vi "integrate_resonance_multifunctional.vi"(0 "integration cluster in":T1, 2 "integration iterations per pixel":u32, 3 "number of pixels":u32, 5 "sampling values in":T2, 7 "choose TAG slice?":bool, 9 "iteration counter in":u32, 11 "pixel counter in":u32, 12 "pick first TAG slice":u32, 13 "pick lastTAG slice":u32, 14 "xy view?":bool) -> (4 "integration cluster out":T1, 6 "iteration counter out":u32, 10 "finished?":bool, 15 "pixel counter out":u32)   [LabVIEW 2010]
uses:
  common_typedefs/channels_cluster.ctl
  integration_cluster.ctl
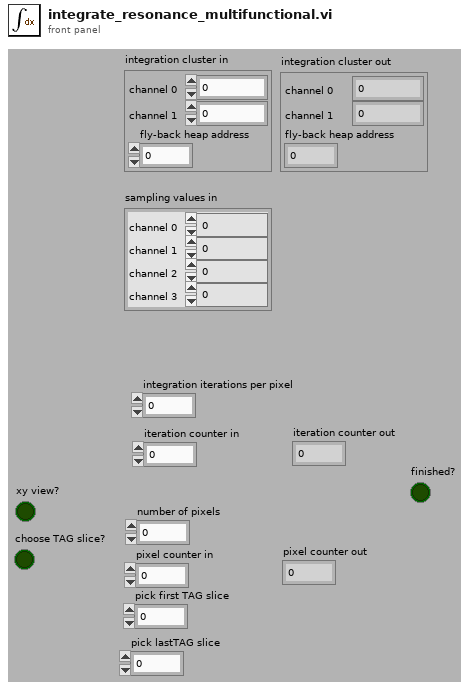
[diagram p1: front panel]
types:
  T1 = typedef "integration_cluster.ctl" = cluster{"channel 0":u32, "channel 1":u32, "fly-back heap address":u32}
  T2 = typedef "channels_cluster.ctl" = cluster{"channel 0":u32, "channel 1":u32, "channel 2":u32, "channel 3":u32}
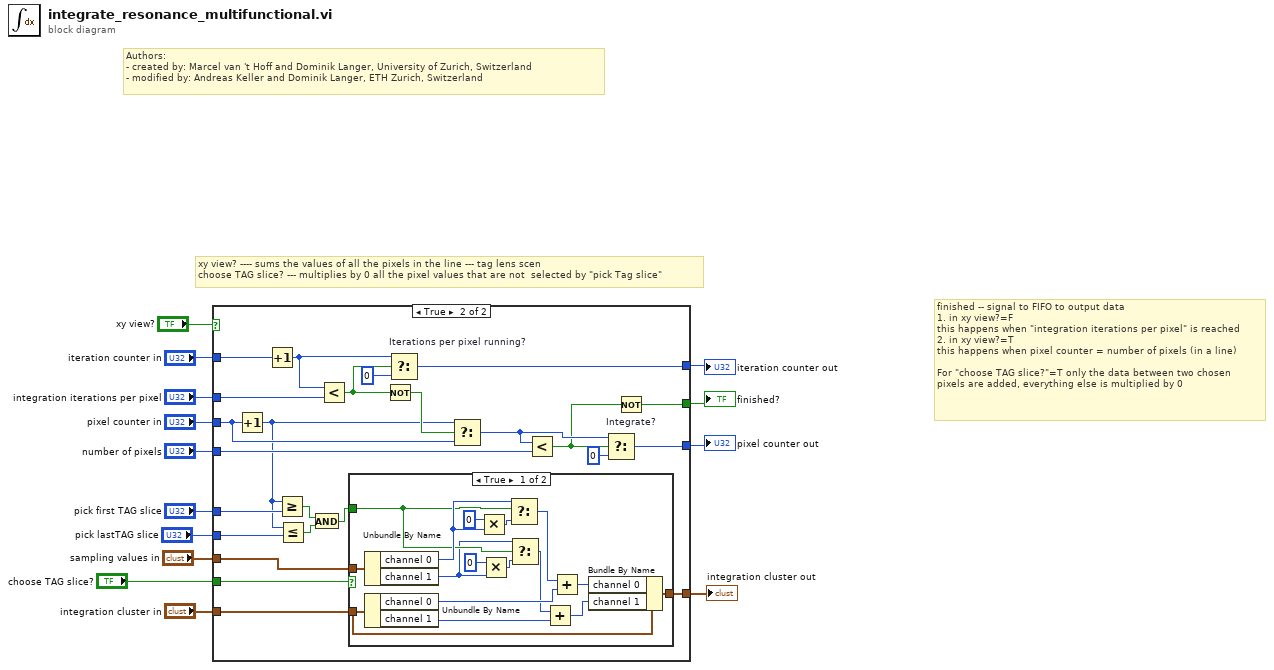
[diagram p0: block diagram]
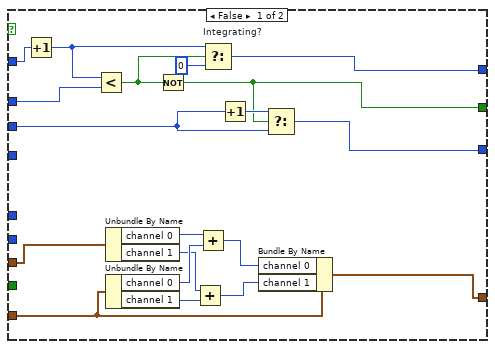
[diagram p2: hidden frame]
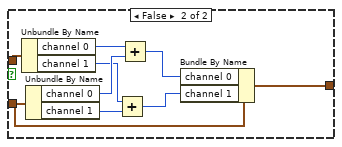
[diagram p3: hidden frame]
diagram:
  # "finished -- signal to FIFO to output data\n1. in xy view?=F\nthis happens when \"integration iterations per pixel\" is reached\n2. in xy view?=T\nthis happens when pixel counter = number of pixels (in a line)\n\nFor \"choose TAG slice?\"=T only the data between two chosen \npixels are added, everything else is multiplied by 0"
  # "xy view? ---- sums the values of all the pixels in the line --- tag lens scen\nchoose TAG slice? --- multiplies by 0 all the pixel values that are not  selected by \"pick Tag slice\""
  # "Authors: \n- created by: Marcel van 't Hoff and Dominik Langer, University of Zurich, Switzerland\n- modified by: Andreas Keller and Dominik Langer, ETH Zurich, Switzerland"
  n1 = case shown="True" "xy view?" {
    tunnel: "sampling values in" -> [w20 w57]
    tunnel: "iteration counter in" -> [w23 w56]
    tunnel: [w15 w53] -> w12
    tunnel: "integration cluster in" -> [w19 w51]
    tunnel: [w18 w50] -> w10
    tunnel: [w16 w42] -> w9
    tunnel: [w17 w44] -> w8
    tunnel: "pixel counter in" -> [w21 w39]
    tunnel: "integration iterations per pixel" -> [w22 w48]
    tunnel: "number of pixels" -> [_ w47]
    tunnel: "pick first TAG slice" -> [_ w41]
    tunnel: "choose TAG slice?" -> [_ w40]
    tunnel: "pick lastTAG slice" -> [_ w34]
    frame False {
      n2 = Increment(x=w23) -> (x+1=w32:u32)
      n3 = Less?(x=w32, y=w22) -> (x < y?=w33:bool)
      n4 = Unbundle By Name(w20) -> ("channel 0"=w29:u32, "channel 1"=w27:u32)
      n5 = Unbundle By Name(w19) -> ("channel 0"=w28:u32, "channel 1"=w26:u32)
      n6 = Not(x=w33) -> (.not. x?=w16:bool)
      n7 = Add(x=w27, y=w26) -> (x+y=w24:u32)
      n8 = Add(x=w29, y=w28) -> (x+y=w25:u32)
      n9 = Select "Integrating?"(t=w32, s=w33, f=u32 0) -> (s? t:f=w15:u32)
      n10 = Increment(x=w21) -> (x+1=w30:u32)
      n11 = Bundle By Name(cluster=w19, "channel 0"=w25, "channel 1"=w24) -> (w18:T1)
      n12 = Select(t=w30, s=w16, f=w21) -> (s? t:f=w17:u32)
    }
    frame True {
      n13 = Increment(x=w39) -> (x+1=w38:u32)
      n14 = Increment(x=w56) -> (x+1=w54:u32)
      n15 = Greater Or Equal?(x=w38, y=w41) -> (x >= y?=w36:bool)
      n16 = Less Or Equal?(x=w38, y=w34) -> (x <= y?=w35:bool)
      n17 = And(x=w36, y=w35) -> (x .and. y?=w37:bool)
      n18 = Less?(x=w54, y=w48) -> (x < y?=w55:bool)
      n19 = case shown="True" w40 {
        tunnel: w57 -> [w70 w82]
        tunnel: w51 -> [w69 w81]
        tunnel: [w68 w80] -> w50
        tunnel: w37 -> [w60 _]
        frame True {
          n20 = Unbundle By Name(w70) -> ("channel 0"=w65:u32, "channel 1"=w58:u32)
          n21 = Unbundle By Name(w69) -> ("channel 0"=w63:u32, "channel 1"=w73:u32)
          n22 = Multiply(x=u32 0, y=w65) -> (x*y=w64:u32)
          n23 = Multiply(x=u32 0, y=w58) -> (x*y=w61:u32)
          n24 = Select(t=w65, s=w60, f=w64) -> (s? t:f=w66:u32)
          n25 = Select(t=w58, s=w60, f=w61) -> (s? t:f=w59:u32)
          n26 = Add(x=w59, y=w73) -> (x+y=w71:u32)
          n27 = Add(x=w66, y=w63) -> (x+y=w72:u32)
          n28 = Bundle By Name(cluster=w69, "channel 0"=w72, "channel 1"=w71) -> (w68:T1)
        }
        frame False {
          n29 = Unbundle By Name(w82) -> ("channel 0"=w79:u32, "channel 1"=w77:u32)
          n30 = Unbundle By Name(w81) -> ("channel 0"=w78:u32, "channel 1"=w76:u32)
          n31 = Add(x=w77, y=w76) -> (x+y=w74:u32)
          n32 = Add(x=w79, y=w78) -> (x+y=w75:u32)
          n33 = Bundle By Name(cluster=w81, "channel 0"=w75, "channel 1"=w74) -> (w80:T1)
        }
      }
      n34 = Not(x=w55) -> (.not. x?=w49:bool)
      n35 = Select "Iterations per pixel running?"(t=w54, s=w55, f=u32 0) -> (s? t:f=w53:u32)
      n36 = Select(t=w38, s=w49, f=w39) -> (s? t:f=w45:u32)
      n37 = Less?(x=w45, y=w47) -> (x < y?=w43:bool)
      n38 = Select "Integrate?"(t=w45, s=w43, f=u32 0) -> (s? t:f=w44:u32)
      n39 = Not(x=w43) -> (.not. x?=w42:bool)
    }
  }
  "finished?" <- w9
  "iteration counter out" <- w12
  "integration cluster out" <- w10
  "pixel counter out" <- w8
